vi "Variant to JSONRPC params.vi"(8 "error in (no error)":errorcluster, 11 "variant":variant) -> (0 "error out":errorcluster, 3 "<JSON>":string)   [LabVIEW 2019, in "JSON-RPC.lvlib"]
uses:
  JSON-RPC.lvlib
  <vilib>/Utility/Data Type/NI_Data Type.lvlib
  <vilib>/JDP Science/JSONtext/JSONtext.lvlib
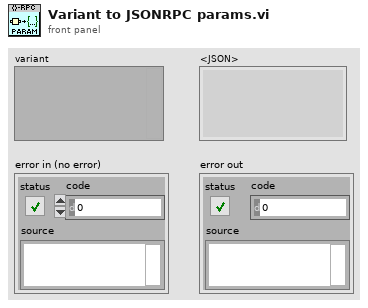
[diagram p1: front panel]
types:
  T1 = typedef "JSONtext.lvlib/JSON Value Type.ctl" = enum16{"Not a JSON Value", "JSON Object", "JSON Array", "String", "Number", "true", "false", "null"}
  T2 = typedef "NI_Data Type.lvlib/Data Type.ctl" = enum8{"Invalid Type", "Void", "I8", "I16", "I32", "I64", "U8", "U16", "U32", "U64", "Single Float", "Double Float", "Extended Float", "Single Complex", "Double Complex", "Extended Complex", "Enum U8", "Enum U16", "Enum U32", "Enum U64", "Single Float With Unit", "Double Float With Unit", "Extended Float With Unit", "Single Complex with Unit", "Double Complex with Unit", "Extended Complex with Unit", "Boolean", "String", "Path", "Picture", "Tag", "Array", "Cluster", "Variant", "LV Variant", "Waveform", "Timestamp", "Digital Waveform", "Digital Data", "ExpressData", "Refnum", "External Data", "VI", "Poly VI", "LabVIEW Class Instance", "Fixed Point", "Set Collection", "Map Collection"}
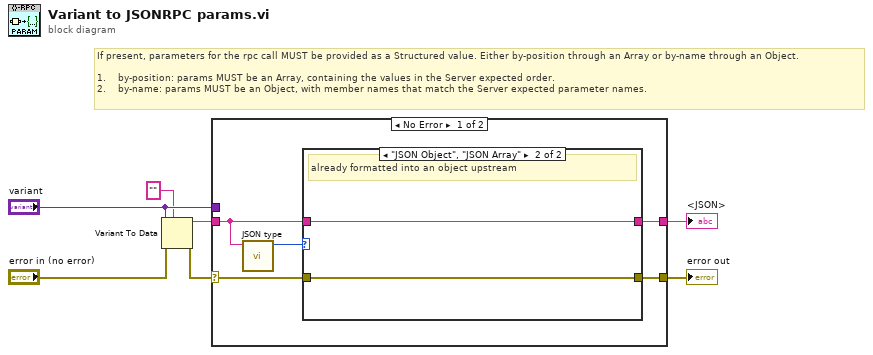
[diagram p0: block diagram]
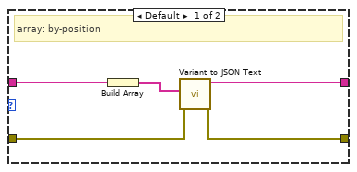
[diagram p2: hidden frame]
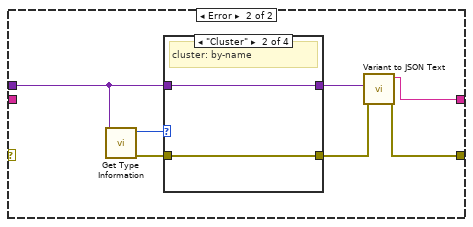
[diagram p3: hidden frame]
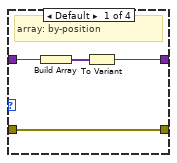
[diagram p4: hidden frame]
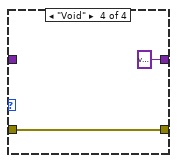
[diagram p6: hidden frame]
diagram:
  # "If present, parameters for the rpc call MUST be provided as a Structured value. Either by-position through an Array or by-name through an Object.\n\n1.    by-position: params MUST be an Array, containing the values in the Server expected order.\n2.    by-name: params MUST be an Object, with member names that match the Server expected parameter names."
  n1 = Variant To Data(error in="error in (no error)", type="", Variant="variant") -> (data=w3:string, error out=w1:errorcluster)
  n2 = case shown="No Error" w1 {
    selector: w1 -> [w9 _]
    tunnel: [w8 w26] -> w7
    tunnel: [w11 w25] -> w6
    tunnel: "variant" -> [_ w24]
    tunnel: w3 -> [w10 _]
    frame No Error {
      n3 = call <vilib>:"JSON type.vi"("JSON"=w10) -> ("JSON Value Type"=w12:T1)  [unwired: 9 in, 1 out]
      n4 = case shown="\"JSON Object\", \"JSON Array\"" w12 {
        tunnel: [w15 w19] -> w11
        tunnel: w10 -> [w17 w19]
        tunnel: w9 -> [w14 w18]
        tunnel: [w13 w18] -> w8
        frame Default {
          # "array: by-position"
          n5 = Build Array(w17) -> (w16:string[])
          n6 = call <vilib>:"Variant to JSON Text.vi"("error in (no error)"=w14, "Variant"=w16) -> ("error out"=w13:errorcluster, "<JSON>"=w15:string)  [unwired: 7 in, 1 out]
        }
        frame "JSON Object", "JSON Array" {
          # "already formatted into an object upstream"
        }
      }
    }
    frame Error {
      n7 = call <vilib>:"Get Type Information.vi"("variant"=w24) -> ("error out"=w21:errorcluster, "type"=w20:T2)  [unwired: 6 in, 3 out]
      n8 = case shown="\"Cluster\"" w20 {
        tunnel: w24 -> [w29 w31 w34 _]
        tunnel: [w28 w31 w34 variant ("params")] -> w22
        tunnel: w21 -> [w27 w32 w33 w35]
        tunnel: [w27 w32 w33 w35] -> w23
        frame Default {
          # "array: by-position"
          n9 = Build Array(w29) -> (w30:variant[])
          n10 = To Variant(anything=w30) -> (Variant=w28:variant)
        }
        frame "Cluster" {
          # "cluster: by-name"
        }
        frame "Array" {
          # "array: by-position"
        }
        frame "Void" {
        }
      }
      n11 = call <vilib>:"Variant to JSON Text.vi"("error in (no error)"=w23, "Variant"=w22) -> ("error out"=w26:errorcluster, "<JSON>"=w25:string)  [unwired: 7 in, 1 out]
    }
  }
  "error out" <- w7
  "<JSON>" <- w6
